vi "Picolog Example Log Temp.vi"() -> ()   [LabVIEW 2016]
uses:
  Controls/Thermocouple.ctl
  Controls/Temperature Units.ctl
panel:
  in  "Tab Control":enum32{"Configuration", "Results", "Dial"}(tab)
  in  "Thermocouples":T1[](array[typedef])=[107, 32, 32, 32, 32, 32, 32, 32, 32, 32] items=["B"=98, "E"=101, "J"=106, "K"=107, "N"=110, "R"=114, "S"=115, "T"=116, "Voltage"=120, "Internal"=0, "Off"=32]
  in  "Mains Frequency":i16(ring) items=["50 Hz", "60 Hz"]
  out "Instrument Handle":i16
  in  "Unit":T2
  in  "Sampling Interval [s]":dbl=0.5 min=0.1 max=100.0 step=0.1 format="%#_13g"
  out "Actual Interval [s]":dbl format="%#_2g"
  out "Temperature\nTable":dbl[](array[numeric]) format="%_4g"
  out "Waveform Chart":waveform(dbl)[](graph)
  out "Temperature":cluster{dbl, dbl}(knob) scale=18.0..40.0
  in  "Stop":bool
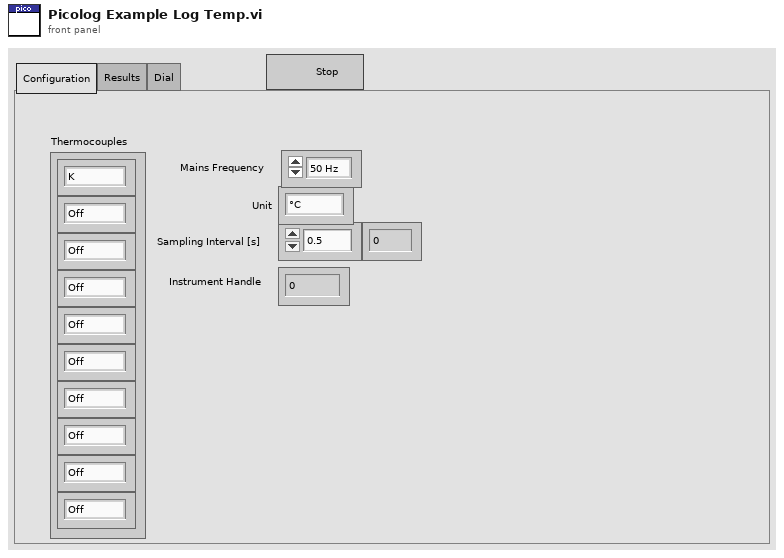
[diagram p1: front panel]
types:
  T1 = typedef "Thermocouple.ctl" = i8
  T2 = typedef "Temperature Units.ctl" = enum16{"°C", "°F", "K", "°R"}
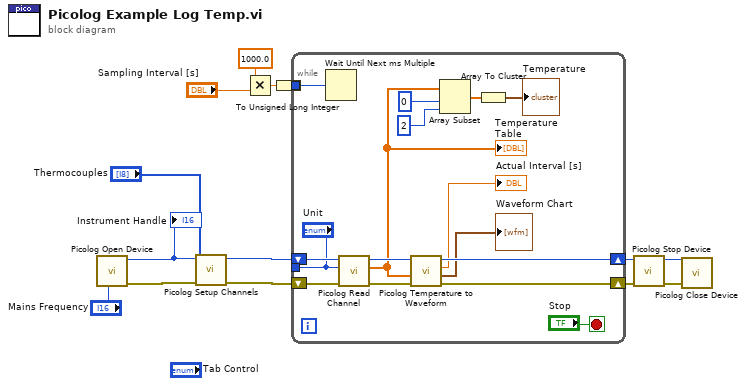
[diagram p0: block diagram]
diagram:
  n1 = call "Picolog Open Device.vi"("Mains Frequency"="Mains Frequency") -> ("Error Out"=w8:errorcluster, "Instrument Handle Out"=w9:i16)  [unwired: 9 in]
  "Instrument Handle" <- w9
  n2 = call "Picolog Setup Channels.vi"("Error In"=w8, "Configurations"="Thermocouples", "Instrument Handle"=w9) -> ("Error Out"=w12:errorcluster, "Instrument Handle Out"=w11:i16)  [unwired: 7 in]
  n3 = Multiply(x=1000.0 ("y"), y="Sampling Interval [s]") -> (x*y=w4:dbl)
  n4 = To Unsigned Long Integer(number=w4) -> (unsigned 32bit integer=w3:u32)
  n5 = while {
    tunnel: ["Unit"] -> _
    shift-right: [w22] -> w10
    shift-left: w12 -> [w28]
    shift-right: [w29] -> w13
    shift-left: w11 -> [w27]
    tunnel: w3 -> [w25]
    stop <- "Stop" stop-if-true
    n6 = Wait Until Next ms Multiple(millisecond multiple=w25) -> ()  [unwired: 1 out]
    n7 = call "Picolog Read Channel.vi"("Error In"=w28, "Units"="Unit", "Instrument Handle In"=w27) -> ("Error Out"=w23:errorcluster, "Temperature buffer"=w20:dbl[], "Instrument Handle Out"=w29:i16)  [unwired: 6 in]
    "Temperature\nTable" <- w20
    n8 = call "Picolog Temperature to Waveform.vi"("Error In"=w23, "Temperature"=w20) -> ("Error Out"=w22:errorcluster, "Temperature Waveform"=→"Waveform Chart":waveform(dbl)[], "Sample Interval [s]"=→"Actual Interval [s]":dbl)  [unwired: 7 in]
    n9 = Array Subset(array=w20, index=0, length=2 ("index")) -> (w17:dbl[])
    n10 = Array To Cluster(array=w17) -> (cluster=→"Temperature":cluster{"[0]":dbl, "[1]":dbl})
  }
  n11 = call "Picolog Stop Device.vi"("Error In"=w10, "Instrument Handle In"=w13) -> ("Error Out"=w6:errorcluster, "Instrument Handle Out"=w14:i16)  [unwired: 8 in]
  n12 = call "Picolog Close Device.vi"("Error In"=w6, "Instrument Handle"=w14) -> ()  [unwired: 9 in, 1 out]
